vi "Source_Funct img viewers names.vi"() -> (1 "Name string: Functional imaging viewer (Rectangles)":string, 3 "Name string: Functional imaging viewer (POI/Mscn)":string)   [LabVIEW 2017]
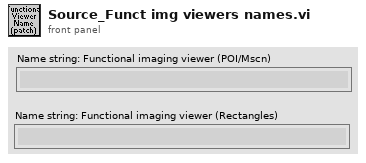
[diagram p1: front panel]
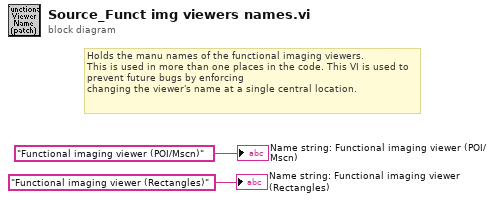
[diagram p0: block diagram]
diagram:
  # "Holds the manu names of the functional imaging viewers.\nThis is used in more than one places in the code. This VI is used to prevent future bugs by enforcing\nchanging the viewer's name at a single central location."
  "Name string: Functional imaging viewer (Rectangles)" <- "Functional imaging viewer (Rectangles)"
  "Name string: Functional imaging viewer (POI/Mscn)" <- "Functional imaging viewer (POI/Mscn)"
